vi "Parent Interfaces.vi"(8 "error in":errorcluster, 10 "Path":path) -> (0 "error out":errorcluster, 2 "Parent Interface Paths":path[](array[path]))   [LabVIEW 2020, in "jettl.lvlib" / "Actor.lvlib" / "Base Actor.lvclass"]
uses:
  Base Actor.lvclass
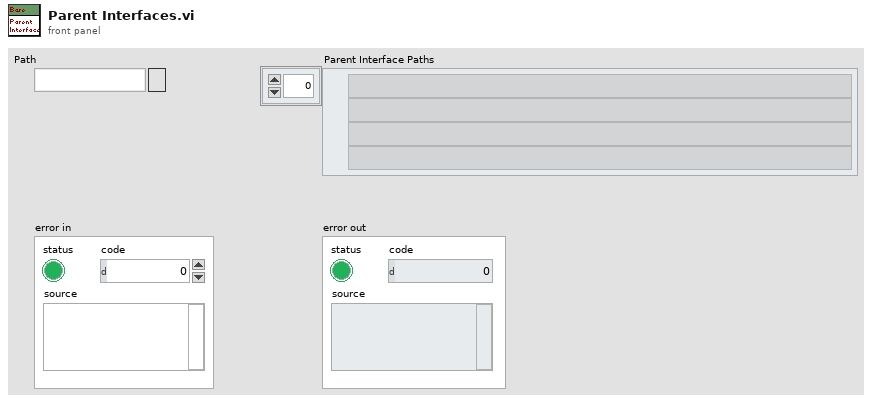
[diagram p1: front panel]
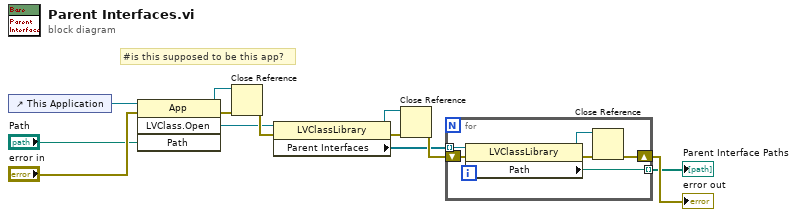
[diagram p0: block diagram]
diagram:
  # "#is this supposed to be this app?"
  n1 = control-ref of="This Application"() -> (w1:refnum<vi>)
  n2 = invoke class="App" method="LVClass.Open"(reference=w1, error in="error in", "Path"="Path") -> (reference out=w13:refnum<vi>, error out=w12:errorcluster, "LVClass.Open"=w10:refnum<vi>)  [unwired: 1 in, 1 out]
  n3 = Close Reference(reference=w13, error in (no error)=w12) -> (error out=w11:errorcluster)
  n4 = property class="LVClassLibrary"(reference=w10, error in=w11) -> (reference out=w8:refnum<vi>, error out=w9:errorcluster, "Parent Interfaces"=w6:refnum<vi>[])
  n5 = Close Reference(reference=w8, error in (no error)=w9) -> (error out=w7:errorcluster)
  n6 = for {
    tunnel: w6 -> [w18] mode=indexing
    shift-right: [w15] -> w5
    shift-left: w7 -> [w19]
    tunnel: [w14] -> w4 mode=indexing
    n7 = property class="LVClassLibrary"(reference=w18, error in=w19) -> (reference out=w16:refnum<vi>, error out=w17:errorcluster, "Path"=w14:path)
    n8 = Close Reference(reference=w16, error in (no error)=w17) -> (error out=w15:errorcluster)
  }
  "error out" <- w5
  "Parent Interface Paths" <- w4
